vi "Search Direction Nodes.vi"(11 "Address":T1) -> (2 "Search Directions":T2[](array[typedef])=[enum."Right", enum."Down", enum."Left", enum."Up"], 3 "Search Direction Nodes":T1[](array[typedef]))   [LabVIEW 2019, in "Grassfire 2D.lvclass"]
uses:
  Grassfire 2D.lvclass
  Node Address--cluster.ctl
  Shared/Direction--enum.ctl
  Shared/Shared.lvlib
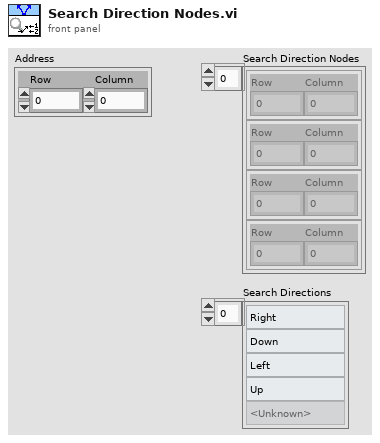
[diagram p1: front panel]
types:
  T1 = typedef "Grassfire 2D.lvclass/Node Address--cluster.ctl" = cluster{"Row":i32, "Column":i32}
  T2 = typedef "Shared.lvlib/Direction--enum.ctl" = enum16{"<Unknown>", "Right", "Down", "Left", "Up"}
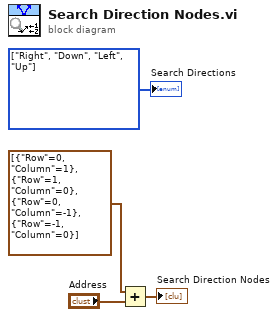
[diagram p0: block diagram]
diagram:
  w3 = T2[] [enum."Right", enum."Down", enum."Left", enum."Up"] items=["<Unknown>", "Right", "Down", "Left", "Up"]
  n1 = Add(x=T1[] [{"Row"=0, "Column"=1}, {"Row"=1, "Column"=0}, {"Row"=0, "Column"=-1}, {"Row"=-1, "Column"=0}], y="Address") -> (x+y=→"Search Direction Nodes":T1[])
  "Search Directions" <- w3
